vi "Create Context.vi"(8 "error in (no error)":errorcluster) -> (0 "error out":errorcluster, 3 "App":refnum<vi>)   [LabVIEW 2020, in "LV-Protoc.lvlib"]
uses:
  LV-Protoc.lvlib
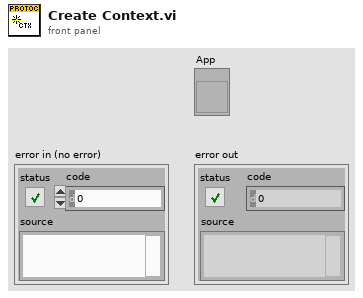
[diagram p1: front panel]
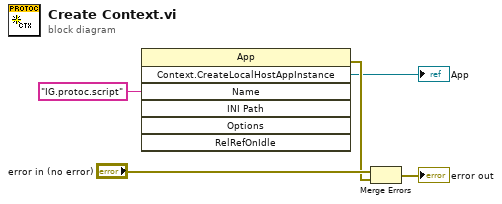
[diagram p0: block diagram]
diagram:
  n1 = invoke class="App" method="Context.CreateLocalHostAppInstance"("Name"="IG.protoc.script" ("Application Instance Name")) -> (error out=w3:errorcluster, "Create Context"=→"App":refnum<vi>)  [unwired: 6 in, 5 out]
  n2 = Merge Errors("error in (no error)", w3) -> (→"error out":errorcluster)
